vi "Compile with Hook.vi"(8 "Error In":errorcluster) -> (0 "Error Out":errorcluster)   [LabVIEW 2018, in "Tests.lvlib" / "Compile.lvlib"]
uses:
  Compile.lvlib
  Support/Mock Compile Hook/Mock Compile Hook.lvclass
  D:/Users/cfield/Code/Field R&D Services/Labstache/src/Toolkit/Hooks/Compile/Process/Process.lvclass
  src/Toolkit/Low-Level/Context/Compiler.lvclass
  Support/Mock Compile Hook/Mock Compile Hook.lvclass/Mock Compile Hook.ctl
  Support/Mock Compile Hook/Read Post.vi
  Support/Mock Compile Hook/Read Pre.vi
  src/Toolkit/Data/Map/Map.lvclass
  D:/Users/cfield/Code/Field R&D Services/Labstache/src/Toolkit/Data/Datum/Datum.lvclass
  src/Toolkit/Data/Map/Support/From String.vi
  src/Toolkit/Support/Compile with Data.vi
  <vilib>/addons/_JKI Toolkits/Caraya/classes/Test/Test.lvclass
  <vilib>/addons/_JKI Toolkits/Caraya/classes/Assert/Assert.lvclass
  src/Toolkit/Toolkit.lvlib
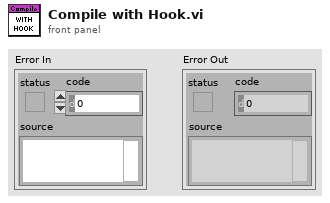
[diagram p1: front panel]
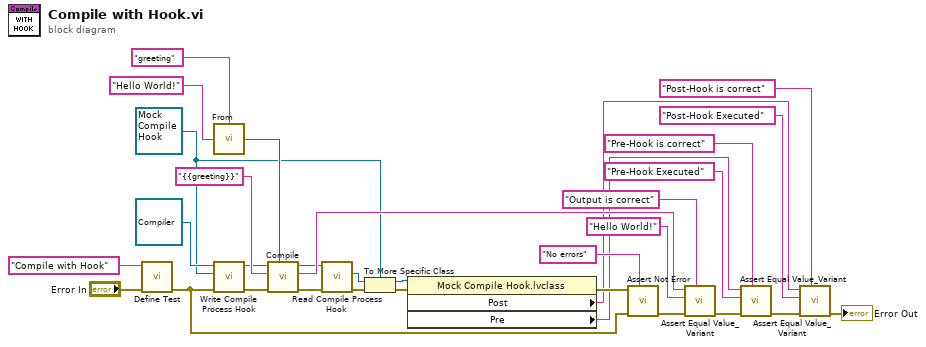
[diagram p0: block diagram]
diagram:
  w2 = refnum<class "Mock Compile Hook.lvclass"> refnum ("Tests.lvlib:Compile.lvlib:Mock Compile Hook.lvclass")
  n1 = call <vilib>:"Define Test.vi"("error in (no error)"="Error In", "Label (VI Title)"="Compile with Hook") -> ("error out"=w4:errorcluster)  [unwired: 9 in]
  n2 = call-poly "From.vi"("Value"="Hello World!", "Key"="greeting") -> ("Map"=w24:refnum<class "Map.lvclass">)
  n3 = call "Write Compile Process Hook.vi"("Error In"=w4, "Compile Process"=w2, "Context In"=refnum<class "Compiler.lvclass"> refnum) -> ("Error Out"=w21:errorcluster, "Context Out"=w20:refnum<class "Compiler.lvclass">)  [unwired: 7 in]
  n4 = call-poly "Compile.vi"("Data"=w24, "Error In"=w21, "Input"="{{greeting}}" ("format string"), "Context In"=w20) -> ("Error Out"=w18:errorcluster, "Output"=w22:string, "Context Out"=w19:refnum<class "Compiler.lvclass">)  [unwired: 5 in]
  n5 = call "Read Compile Process Hook.vi"("Error In"=w18, "Context In"=w19) -> ("Error Out"=w12:errorcluster, "Compile Process"=w1:refnum<class "Process.lvclass">)  [unwired: 7 in, 1 out]
  n6 = To More Specific Class(target class=w2, reference=w1, error in=w12) -> (specific class reference=w9:refnum<class "Mock Compile Hook.lvclass">, error out=w10:errorcluster)
  n7 = property class="Mock Compile Hook.lvclass"(reference=w9, error in=w10) -> (error out=w11:errorcluster, "Post"=w8:string, "Pre"=w7:string)  [unwired: 1 out]
  n8 = call <vilib>:"Assert Not Error.vi"("Label"="No errors", "error in (no error)"=w4, "Not Error?"=w11) -> ("error out"=w29:errorcluster)  [unwired: 8 in]
  n9 = call <vilib>:"Assert Equal Value_Variant.vi"("Label"="Output is correct", "error in (no error)"=w29, "Y"="Hello World!" ("Value"), "X"=w22) -> ("error out"=w17:errorcluster)  [unwired: 7 in]
  n10 = call <vilib>:"Assert Equal Value_Variant.vi"("Label"="Pre-Hook is correct", "error in (no error)"=w17, "Y"="Pre-Hook Executed" ("Post"), "X"=w7) -> ("error out"=w16:errorcluster)  [unwired: 7 in]
  n11 = call <vilib>:"Assert Equal Value_Variant.vi"("Label"="Post-Hook is correct", "error in (no error)"=w16, "Y"="Post-Hook Executed" ("Post"), "X"=w8) -> ("error out"=→"Error Out":errorcluster)  [unwired: 7 in]
